vi "AddressRef.vi"(7 "Init":bool, 10 "add_type in":refnum<vi>) -> (2 "add_type out":refnum<vi>)   [LabVIEW 2017]
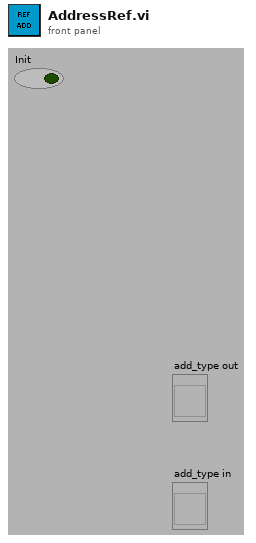
[diagram p1: front panel]
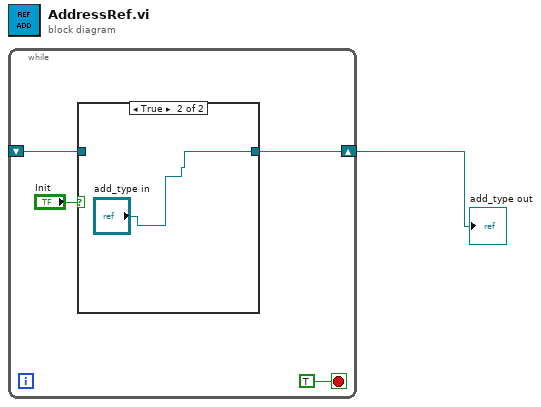
[diagram p0: block diagram]
diagram:
  n1 = while {
    shift-right: [w4] -> w1
    shift-left: _ -> [w2]
    stop <- TRUE stop-if-true
    n2 = case shown="True" "Init" {
      tunnel: [w6 "add_type in"] -> w4
      tunnel: w2 -> [w6 _]
      frame False {
      }
      frame True {
      }
    }
  }
  "add_type out" <- w1
